vi "RotatePolys.vi"(8 "Angle":sgl, 11 "Polys":T1[](array[typedef])) -> (3 "RotatedPolys":cluster{cluster{sgl, sgl, "Slope":dbl}[]}[](array[cluster]))   [LabVIEW 2014]
uses:
  TypeDefs/Poly2DwSlope.ctl
  TypeDefs/Point2DwSlope.ctl
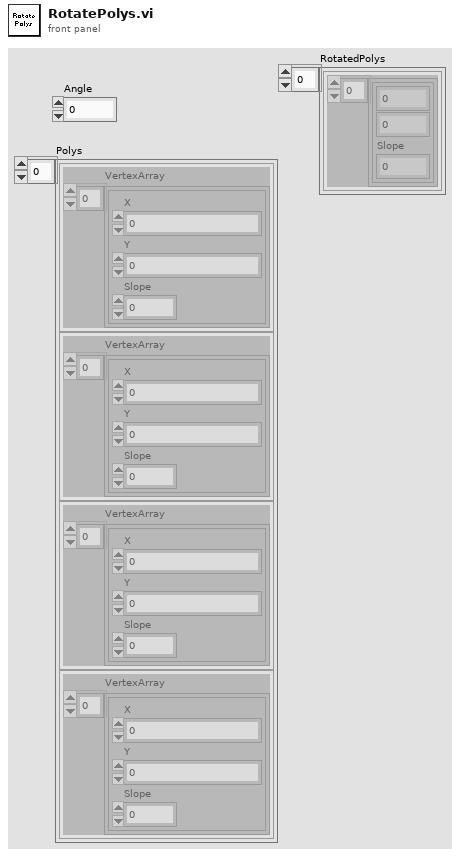
[diagram p1: front panel]
types:
  T1 = typedef "Poly2DwSlope.ctl" = cluster{"VertexArray":T2[]}
  T2 = typedef "Point2DwSlope.ctl" = cluster{"X":sgl, "Y":sgl, "Slope":dbl}
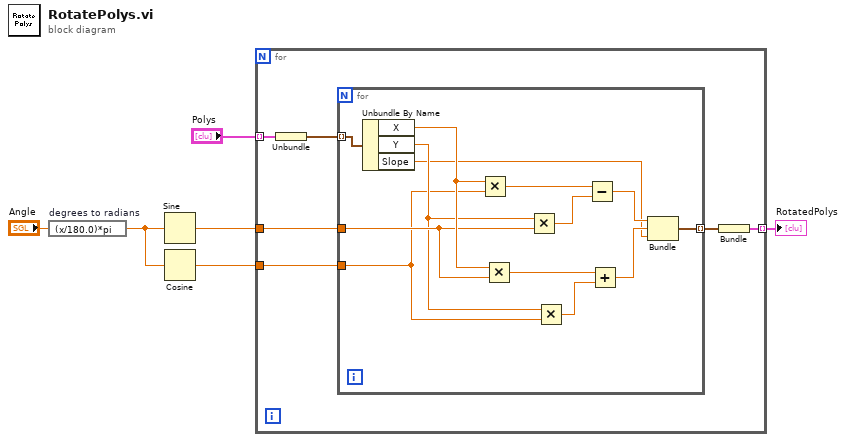
[diagram p0: block diagram]
diagram:
  n1 = expression code="(x/180.0)*pi" "degrees to radians"("Angle") -> (w5:sgl)
  n2 = Sine(x=w5) -> (sin(x)=w3:sgl)
  n3 = Cosine(x=w5) -> (cos(x)=w2:sgl)
  n4 = for {
    tunnel: "Polys" -> [w12] mode=indexing
    tunnel: w3 -> [w10]
    tunnel: w2 -> [w9]
    tunnel: [w7] -> w1 mode=indexing
    n5 = Unbundle(w12) -> ("VertexArray"=w11:T2[])
    n6 = for {
      tunnel: w11 -> [w25] mode=indexing
      tunnel: w10 -> [w21]
      tunnel: w9 -> [w18]
      tunnel: [w14] -> w8 mode=indexing
      n7 = Unbundle By Name(w25) -> ("X"=w22:sgl, "Y"=w19:sgl, "Slope"=w13:dbl)
      n8 = Multiply(x=w22, y=w18) -> (x*y=w24:sgl)
      n9 = Multiply(x=w22, y=w21) -> (x*y=w20:sgl)
      n10 = Multiply(x=w19, y=w21) -> (x*y=w23:sgl)
      n11 = Multiply(x=w19, y=w18) -> (x*y=w17:sgl)
      n12 = Subtract(x=w24, y=w23) -> (x-y=w16:sgl)
      n13 = Add(x=w20, y=w17) -> (x+y=w15:sgl)
      n14 = Bundle(w16, w15, "Slope"=w13) -> (w14:cluster{sgl, sgl, "Slope":dbl})  [unwired: 1 in]
    }
    n15 = Bundle(w8) -> (w7:cluster{cluster{sgl, sgl, "Slope":dbl}[]})  [unwired: 1 in]
  }
  "RotatedPolys" <- w1
